vi "Listen for Interrupt.vi"(8 "error in (no error)":errorcluster, 10 "Response Msg in":refnum<class "Response Msg.lvclass">, 11 "Response Core in":refnum<class "Interruptible Reply Core.lvclass">) -> (0 "error out":errorcluster, 2 "Response Msg out":refnum<class "Response Msg.lvclass">, 3 "Response Core out":refnum<class "Interruptible Reply Core.lvclass">)   [LabVIEW 2020, in "Publisher.lvlib" / "Interruptible Reply Core.lvclass"]
doc: "Await interrupt in parallel with recieve to enable termination of Recieve.\n\nThis implementation awaits interrupt on the Interrupt Notifier. On interrupt, timeout or error the Message is dropped."
uses:
  Interruptible Reply Core.lvclass
  Response Msg.lvclass
  Interruptible Reply Core.lvclass/Interruptible Reply Core.ctl
  PPL/HDH.Data.Generic.lvlibp/Synchronization/Notifier/Notifier.lvclass
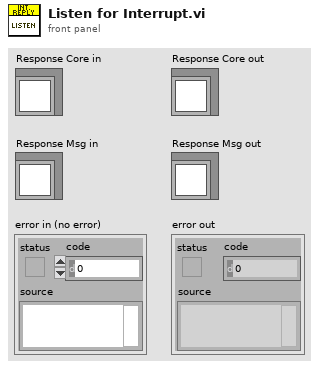
[diagram p1: front panel]
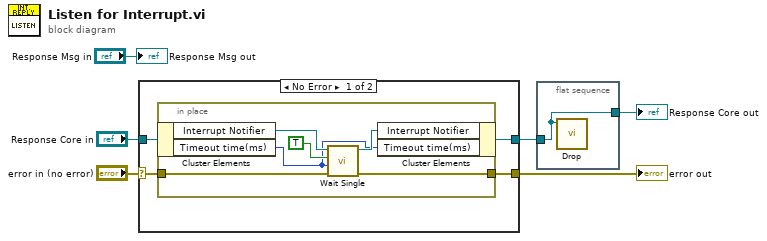
[diagram p0: block diagram]
diagram:
  n1 = case shown="No Error" "error in (no error)" {
    selector: "error in (no error)" -> [w9 w18]
    tunnel: [w7 w18] -> w4
    tunnel: [w8 w17] -> w2
    tunnel: "Response Core in" -> [w10 w17]
    frame No Error {
      n2 = in-place {
        in-place-border: w9 -> [w14]
        in-place-border: [w11] -> w7
        n3 = in-place-cluster #1(w10) -> ("Interrupt Notifier"=w16:refnum<class "Notifier.lvclass">, "Timeout time(ms)"=w12:i32)
        n4 = call "Wait Single.vi"("error in (no error)"=w14, "Timeout in ms (-1)"=w12, "Ignore previous (F)"=TRUE, "Notifier in"=w16) -> ("error out"=w11:errorcluster, "Notifier out"=w13:refnum<class "Notifier.lvclass">)  [unwired: 4 in, 2 out]
        n5 = in-place-cluster #1("Interrupt Notifier"=w13, "Timeout time(ms)"=w12) -> (w8:refnum<class "Interruptible Reply Core.lvclass">)
      }
    }
    frame Error {
    }
  }
  "error out" <- w4
  n6 = flat-sequence {
    tunnel: [w19] -> w3
    tunnel: w2 -> [w19]
    frame #0 {
      n7 = call-dynamic "Drop.vi"("Response Core in"=w19) -> ()  [unwired: 11 in]
    }
  }
  "Response Core out" <- w3
  "Response Msg out" <- "Response Msg in"
